vi "AddOpenCircuitPotential.vi"(0 "deviceName":string, 1 "maxDuration":sgl=1.0, 2 "minVoltage":sgl=-inf, 3 "approxMaxVoltage":sgl=inf, 5 "channel":u8, 7 "repeats":u16=1, 9 "samplingInterval":sgl=1.0, 11 "error in (no error)":errorcluster, 12 "maxVoltage":sgl=inf, 13 "mindVdt":sgl, 14 "isAutoVoltageRange":bool=TRUE) -> (15 "error out":errorcluster)   [LabVIEW 2018]
doc: "EXPORT void AisAddOpenCircuitPotential(const char* deviceName, uint8_t channel, uint16_t repeats, float samplingInterval, float maxDuration, float maxVoltage, float minVoltage, float mindVdt, float approxMaxVoltage, bool isAutoVoltageRange);"
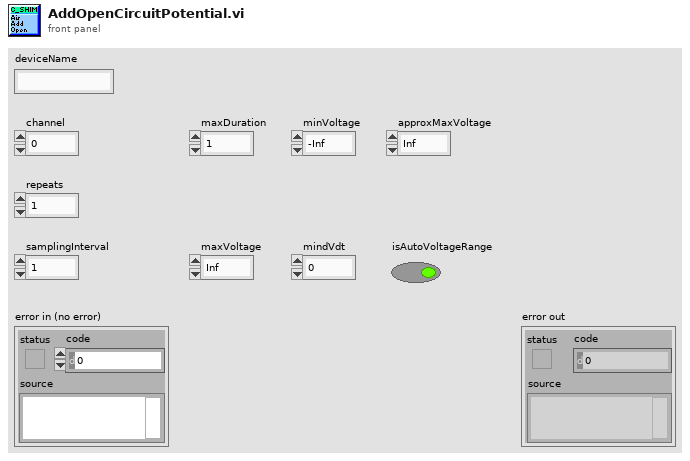
[diagram p1: front panel]
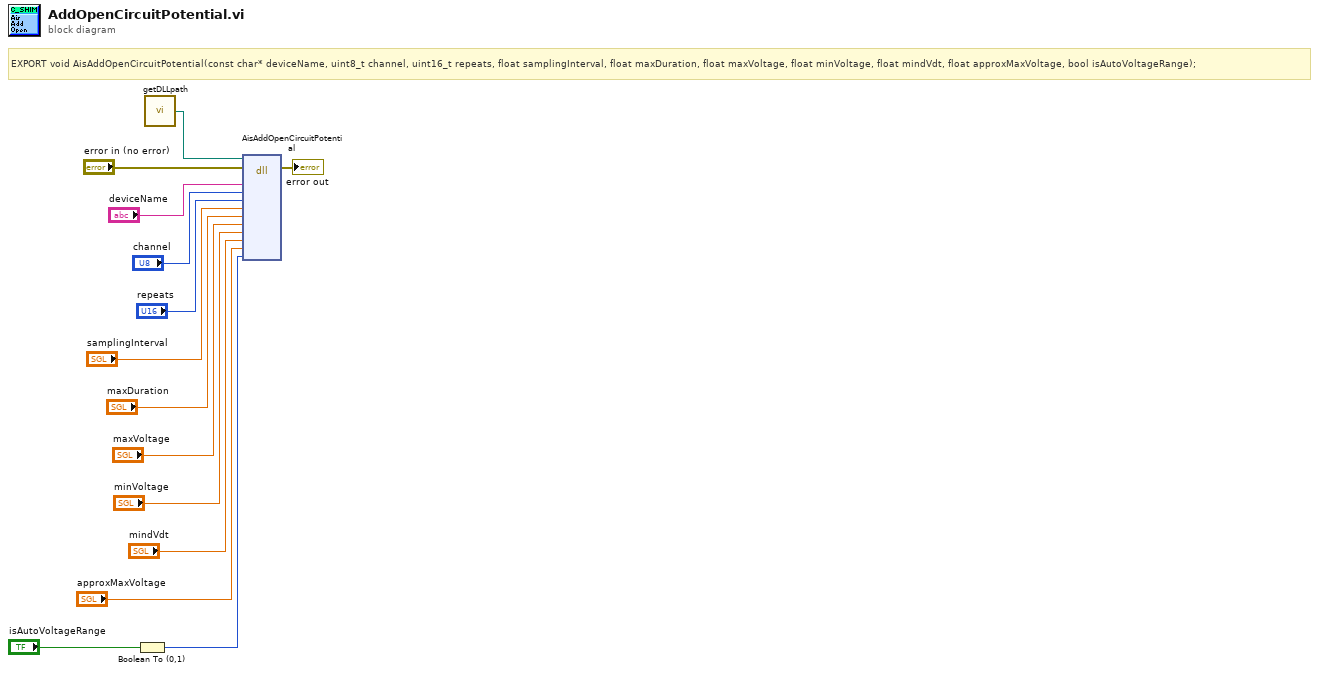
[diagram p0: block diagram]
diagram:
  # "EXPORT void AisAddOpenCircuitPotential(const char* deviceName, uint8_t channel, uint16_t repeats, float samplingInterval, float maxDuration, float maxVoltage, float minVoltage, float mindVdt, float approxMaxVoltage, bool isAutoVoltageRange);"
  n1 = Boolean To (0,1)(Boolean="isAutoVoltageRange") -> (0, 1=w4:i16)
  n2 = call "getDLLpath.vi"() -> ("DLL_Path"=w1:path)
  n3 = dll-call lib="?" fn="AisAddOpenCircuitPotential"(path in=w1, error in="error in (no error)", "deviceName"="deviceName", "channel"="channel", "repeats"="repeats", "samplingInterval"="samplingInterval", "maxDuration"="maxDuration", "maxVoltage"="maxVoltage", "minVoltage"="minVoltage", "mindVdt"="mindVdt", "approxMaxVoltage"="approxMaxVoltage", "isAutoVoltageRange"=w4) -> (error out=→"error out":errorcluster)  [unwired: 12 in, 1 out]
